vi "Measure.vi"(8 "error in (no error)":errorcluster caption="错误输入（无错误）", 11 "Fluke 8808A 输入":refnum<class "Fluke 8808A.lvclass">) -> (0 "error out":errorcluster caption="错误输出", 2 "Measurement":dbl, 3 "Fluke 8808A 输出":refnum<class "Fluke 8808A.lvclass">)   [LabVIEW 2020, in "Fluke 8808A.lvlib" / "Fluke 8808A.lvclass"]
uses:
  Fluke 8808A.lvclass
  <instrlib>/Fluke 8808/Fluke 8808.lvlib
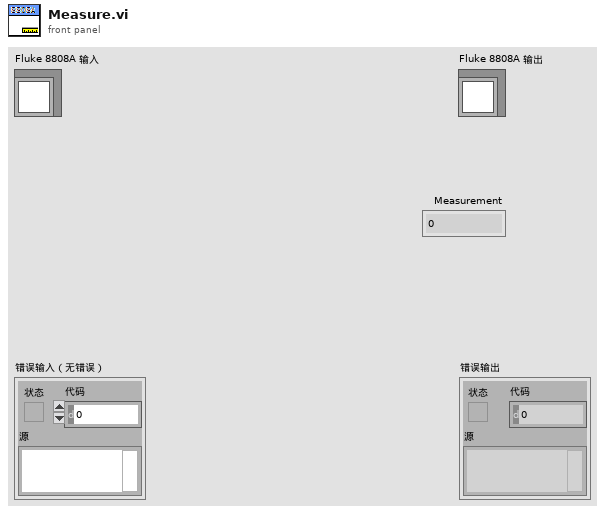
[diagram p1: front panel]
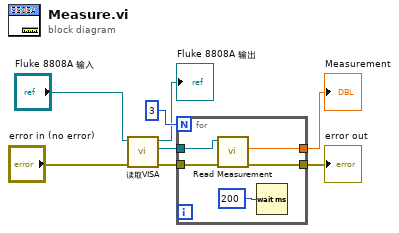
[diagram p0: block diagram]
diagram:
  n1 = call "读取VISA.vi"("error in (no error)"="error in (no error)", "数字多用表接口输入"="Fluke 8808A 输入") -> ("error out"=w5:errorcluster, "VISA"=w7:refnum<visa-resource-name>, "数字多用表接口输出"=→"Fluke 8808A 输出":refnum<class "Fluke 8808A.lvclass">)  [unwired: 7 in]
  n2 = for {
    N: 3 -> [_]
    tunnel: w7 -> [w13]
    tunnel: w5 -> [w12]
    tunnel: [w11] -> w3
    tunnel: [w10] -> w2
    n3 = call <instrlib>:"Read Measurement.vi"("error in (no error)"=w12, "VISA resource name"=w13) -> ("error out"=w11:errorcluster, "Primary Display Measurement"=w10:dbl)  [unwired: 4 in, 4 out]
    n4 = Wait (ms)(milliseconds to wait=u32 200 ("等待时间（毫秒）")) -> ()  [unwired: 1 out]
  }
  "error out" <- w3
  "Measurement" <- w2
